vi "integrateCameraEvents.vi"(8 "error in (no error)":errorcluster, 11 "CameraManager in":refnum<class "CameraManager.lvclass">) -> (0 "error out":errorcluster, 3 "CameraManager out":refnum<class "CameraManager.lvclass">)   [LabVIEW 2011, in "iManagement.lvlib" / "CameraManager.lvclass"]
uses:
  CameraManager.lvclass
  CameraManager.lvclass/CameraManager.ctl
  Hal/Channels/Camera/CameraController.lvclass
  Hal/Channels/Camera/CameraEventsManager/CameraEventsManger.lvclass
  Tools/Filing/FileNeologist/FileNeologist.lvclass
  Tools/Filing.lvlib
  Tools/ImageProcessor/BECImageProcessor.lvclass
panel:
  in  "generate error":bool
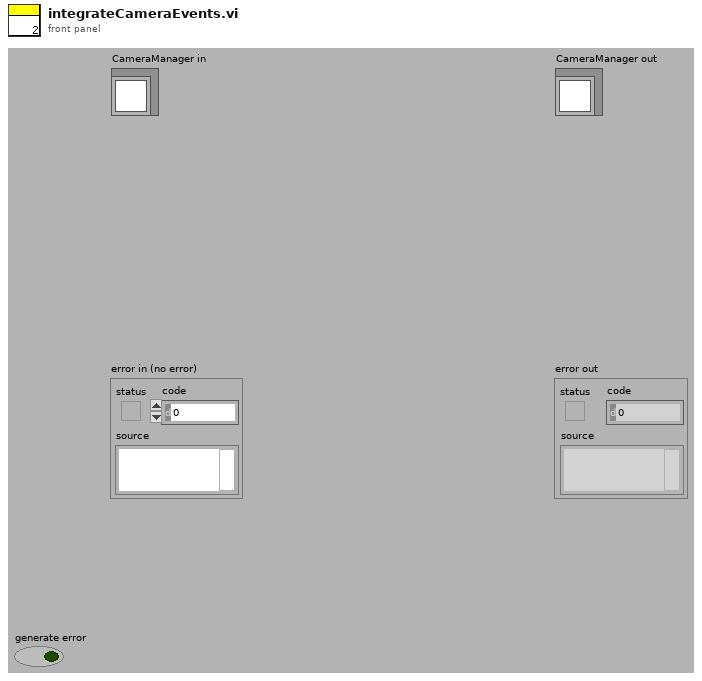
[diagram p1: front panel]
types:
  T1 = cluster{"loadCameraSettingsEvent":refnum<user-event>}
  T2 = cluster{"settingsFrontEndEvents":cluster{"loadSettingsFromPath":refnum<user-event>, "lookUpElementEvent":refnum<user-event>, "saveSettings":refnum<user-event>, "loadSettings":refnum<user-event>, "close":refnum<user-event>, "replaceElement":refnum<user-event>, "findParentNodes":refnum<user-event>, "createNode":refnum<user-event>}, "settingBackEndEvents":cluster{"defaultSettingsPathRequest":refnum<user-event>, "searchResultEvent":refnum<user-event>, "settingsSaved":refnum<user-event>, "settingsLoaded":refnum<user-event>, "foundParentNode":refnum<user-event>}}
  T3 = cluster{"frontEndEvents":cluster{"snapShotEvent":refnum<user-event>, "stopShooting":refnum<user-event>, "userSnapShot":refnum<user-event>}, "backEndEvents":cluster{"picture":refnum<user-event>}}
  T4 = cluster{"snapShotEvent":refnum<user-event>, "stopShooting":refnum<user-event>, "userSnapShot":refnum<user-event>}
  T5 = cluster{"loadSettingsFromPath":refnum<user-event>, "lookUpElementEvent":refnum<user-event>, "saveSettings":refnum<user-event>, "loadSettings":refnum<user-event>, "close":refnum<user-event>, "replaceElement":refnum<user-event>, "findParentNodes":refnum<user-event>, "createNode":refnum<user-event>}
  T6 = cluster{"closeEvent":refnum<user-event>, "temperatureUpdateEvent":refnum<user-event>, "displayErrorEvent":refnum<user-event>, "setPointUpdateEvent":refnum<user-event>}
  T7 = cluster{"Path":path, "atomNumber":dbl, " cloudWidth x":dbl, " cloudWidth z":dbl}
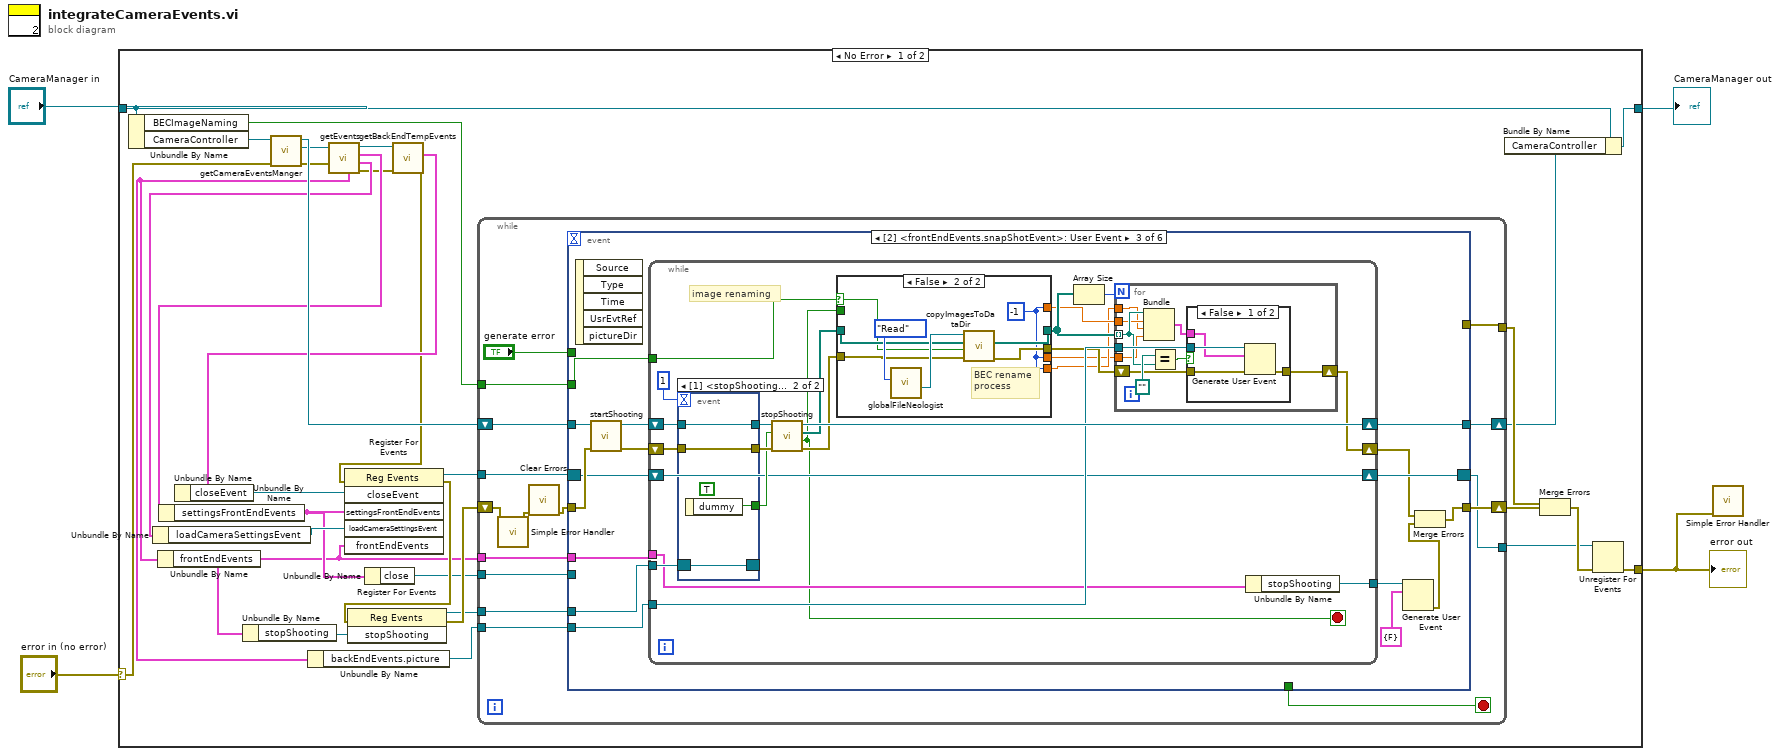
[diagram p0: block diagram]
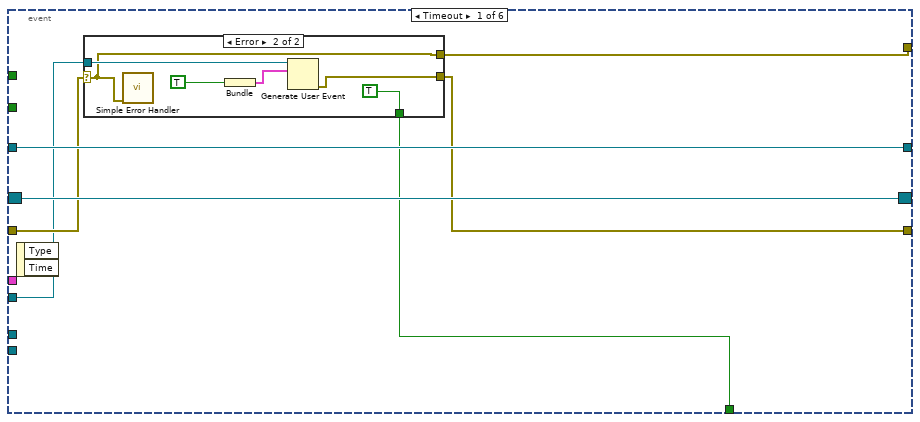
[diagram p2: hidden frame]
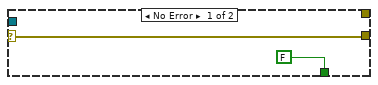
[diagram p3: hidden frame]
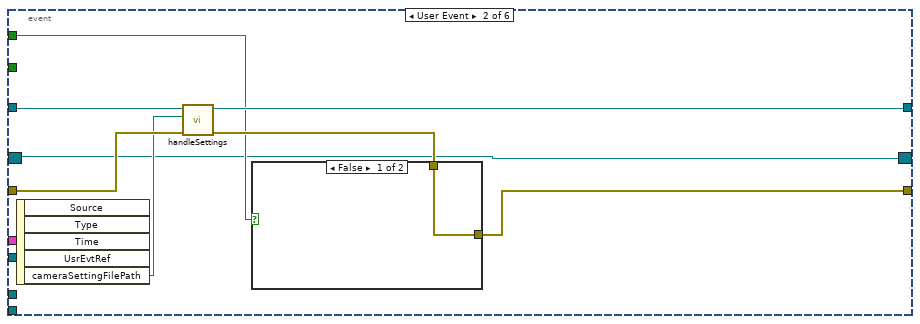
[diagram p4: hidden frame]
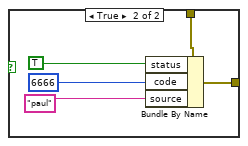
[diagram p5: hidden frame]
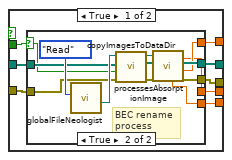
[diagram p6: hidden frame]
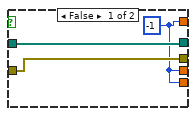
[diagram p7: hidden frame]
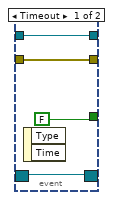
[diagram p9: hidden frame]
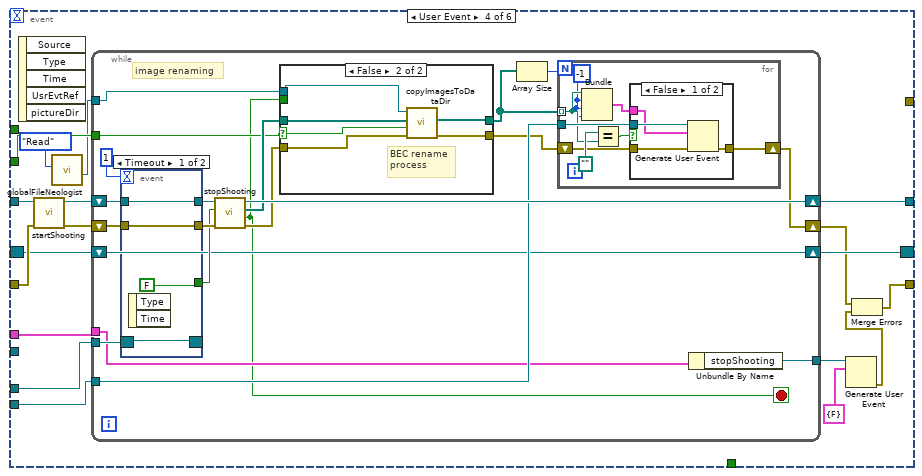
[diagram p10: hidden frame]
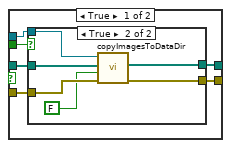
[diagram p11: hidden frame]
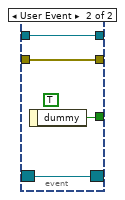
[diagram p14: hidden frame]
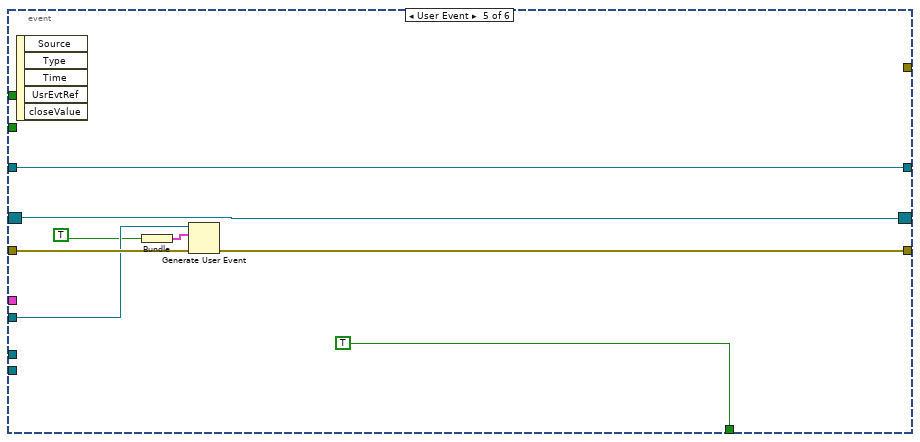
[diagram p15: hidden frame]
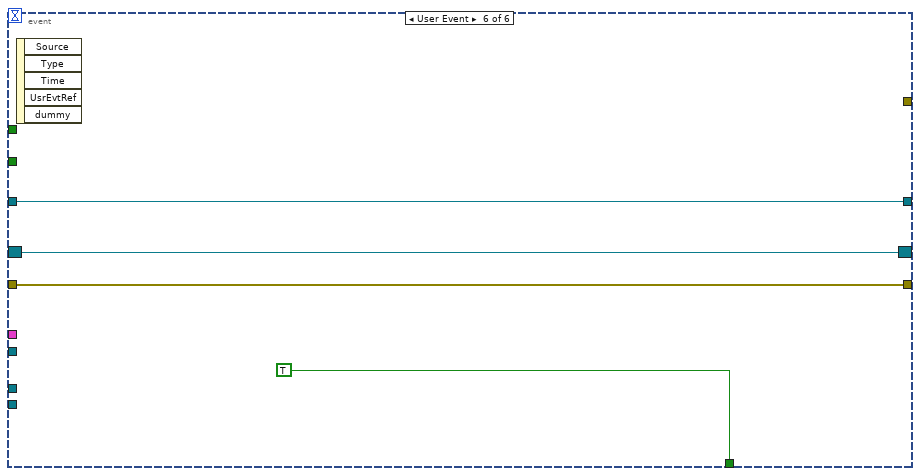
[diagram p16: hidden frame]
diagram:
  n1 = case shown="No Error" "error in (no error)" {
    selector: "error in (no error)" -> [w36 w268]
    tunnel: [w6 w268] -> w1
    tunnel: [w7 w267] -> w2
    tunnel: "CameraManager in" -> [w9 w267]
    frame No Error {
      n2 = Unbundle By Name(w9) -> ("BECImageNaming"=w5:bool, "CameraController"=w35:refnum<class "CameraController.lvclass">)
      n3 = call-dynamic "getCameraEventsManger.vi"("error in (no error)"=w36, "CameraController.lvclass in"=w35) -> ("error out"=w32:errorcluster, "Hardware:Channels.lvlib:CameraEventsManger.lvclass"=w33:refnum<class "CameraEventsManger.lvclass">, "CameraController.lvclass out"=w34:refnum<class "CameraController.lvclass">)  [unwired: 7 in]
      n4 = call-dynamic "getEvents.vi"("error in (no error)"=w32, "CameraEventsManger in"=w33) -> ("error out"=w26:errorcluster, "cameraSettingsEventsRef"=w30:T1, "settingsEvents"=w31:T2, "CameraEventsManger out"=w27:refnum<class "CameraEventsManger.lvclass">, "snapperEvents"=w17:T3)  [unwired: 5 in]
      n5 = Unbundle By Name(w30) -> ("loadCameraSettingsEvent"=w29:refnum<user-event>)
      n6 = Unbundle By Name(w17) -> ("frontEndEvents"=w8:T4)
      n7 = Unbundle By Name(w31) -> ("settingsFrontEndEvents"=w18:T5)
      n8 = Unbundle By Name(w8) -> ("stopShooting"=w28:refnum<user-event>)
      n9 = Unbundle By Name(w17) -> ("backEndEvents.picture"=w16:refnum<user-event>)
      n10 = Unbundle By Name(w18) -> ("close"=w20:refnum<user-event>)
      n11 = call-dynamic "getBackEndTempEvents.vi"("error in (no error)"=w26, "CameraEventsManger.lvclass in"=w27) -> ("error out"=w15:errorcluster, "backEndTempEvents"=w25:T6)  [unwired: 7 in, 1 out]
      n12 = Unbundle By Name(w25) -> ("closeEvent"=w24:refnum<user-event>)
      n13 = register-events(error in=w15, w24, w18, w29, w8) -> (reference out=w23:refnum<event-registration>, error out=w22:errorcluster)  [unwired: 1 in]
      n14 = register-events(error in=w22, w28) -> (reference out=w19:refnum<event-registration>, error out=w21:errorcluster)  [unwired: 1 in]
      n15 = while {
        tunnel: w23 -> [w52]
        shift-right: [w49] -> w10
        shift-left: w34 -> [w50]
        shift-right: [w48] -> w13
        shift-left: w21 -> [w39]
        tunnel: [w47] -> w11
        tunnel: w16 -> [w42]
        tunnel: w19 -> [w46]
        tunnel: w20 -> [w45]
        tunnel: [w44] -> w14
        tunnel: w8 -> [w41]
        tunnel: w5 -> [w40]
        stop <- w51 stop-if-true
        n16 = call <vilib>:"Simple Error Handler.vi"("error in (no error)"=w39) -> ("error out"=w38:errorcluster)  [unwired: 4 in, 4 out]
        n17 = call <vilib>:"Clear Errors.vi"("error in (no error)"=w38) -> ("error out"=w37:errorcluster)  [unwired: 6 in]
        n18 = event shown="[2] <frontEndEvents.snapShotEvent>: User Event" {
          selector: w52 -> [w58 w68 w95 w190 w259 w265]
          dyn-events: [w58 w68 w92 w187 w259 w265] -> w47
          timeout: _ -> [_ _ _ _ _ _]
          tunnel: [w53 _ _ _ TRUE TRUE] -> w51
          tunnel: w50 -> [w59 w75 w97 w192 w262 w264]
          tunnel: [w59 w74 w91 w186 w262 w264] -> w49
          tunnel: w37 -> [w57 w73 w96 w191 w260 w263]
          tunnel: [w56 w70 w84 w175 w261 w263] -> w48
          tunnel: w42 -> [_ _ w90 w185 _ _]
          tunnel: w46 -> [_ _ w89 w184 _ _]
          tunnel: w45 -> [w55 _ _ _ w258 _]
          tunnel: [w54 _ _ _ _ _] -> w44
          tunnel: "generate error" -> [_ w69 _ _ _ _]
          tunnel: w41 -> [_ _ w88 w183 _ _]
          tunnel: w40 -> [_ _ w85 w180 _ _]
          event Timeout {
            n19 = event-data() -> ()  [unwired: 1 in, 2 out]
            n20 = case shown="Error" w57 {
              selector: w57 -> [w61 w62]
              tunnel: [w61 w64] -> w56
              tunnel: w55 -> [_ w65]
              tunnel: [_ w62] -> w54
              tunnel: [FALSE TRUE] -> w53
              frame No Error {
              }
              frame Error {
                n21 = call <vilib>:"Simple Error Handler.vi"("error in (no error)"=w62) -> ()  [unwired: 4 in, 5 out]
                n22 = Bundle(TRUE) -> (w66:cluster{bool})  [unwired: 1 in]
                n23 = Generate User Event(user event=w65, event data cluster=w66) -> (error out=w64:errorcluster)  [unwired: 1 in, 1 out]
              }
            }
          }
          event User Event {
            n24 = event-data() -> ("cameraSettingFilePath"=w72:path)  [unwired: 1 in, 4 out]
            n25 = call-dynamic "handleSettings.vi"("error in (no error)"=w73, "Path"=w72, "CameraController in"=w75) -> ("error out"=w71:errorcluster, "CameraController out"=w74:refnum<class "CameraController.lvclass">)  [unwired: 7 in]
            n26 = case shown="False" w69 {
              tunnel: w71 -> [w76 w81]
              tunnel: [w76 w77] -> w70
              frame False {
              }
              frame True {
                n27 = Bundle By Name(cluster=w81, "status"=TRUE, "code"=6666, "source"="paul") -> (w77:errorcluster)
              }
            }
          }
          event User Event {
            n28 = event-data() -> ()  [unwired: 1 in, 5 out]
            n29 = call-dynamic "startShooting.vi"("error in (no error)"=w96, "CameraController in"=w97) -> ("error out"=w93:errorcluster, "CameraController out"=w94:refnum<class "CameraController.lvclass">)  [unwired: 6 in, 2 out]
            n30 = while {
              shift-right: [w119] -> w91
              shift-left: w94 -> [w120]
              shift-right: [w109] -> w83
              shift-left: w93 -> [w117]
              shift-right: [w111] -> w92
              shift-left: w95 -> [w111]
              tunnel: w90 -> [w113]
              tunnel: w89 -> [w112]
              tunnel: w88 -> [w110]
              tunnel: [w108] -> w87
              tunnel: w85 -> [w102]
              stop <- w101 stop-if-true
              # "image renaming"
              n31 = event shown="[1] <stopShooting>: User Event" {
                selector: w112 -> [w170 w172]
                dyn-events: [w170 w172] -> _
                timeout: 1 -> [_ _]
                tunnel: [w169 w174] -> w118
                tunnel: w120 -> [w169 w174]
                tunnel: w117 -> [w168 w173]
                tunnel: [w168 w173] -> w116
                tunnel: [FALSE w171] -> w114
                event Timeout {
                  n32 = event-data() -> ()  [unwired: 1 in, 2 out]
                }
                event User Event {
                  (unwired) TRUE
                  n33 = event-data() -> ("dummy"=w171:bool)  [unwired: 1 in]
                }
              }
              n34 = call-dynamic "stopShooting.vi"("error in (no error)"=w116, "stop"=w114, "CameraController in"=w118) -> ("error out"=w104:errorcluster, "Stopped"=w101:bool, "Array"=w106:path[], "CameraController out"=w119:refnum<class "CameraController.lvclass">)  [unwired: 5 in]
              n35 = case shown="False" w102 {
                selector: w102 -> [_ w145]
                tunnel: w106 -> [w128 w149]
                tunnel: [w125 w146] -> w105
                tunnel: w104 -> [w127 w148]
                tunnel: [w126 w147] -> w103
                tunnel: w101 -> [w124 _]
                tunnel: [w123 w144] -> w100
                tunnel: [w122 w144] -> w99
                tunnel: [w121 w144] -> w98
                frame True {
                  n36 = case shown="True" w124 {
                    selector: w124 -> [_ w140]
                    tunnel: w128 -> [w131 w141]
                    tunnel: w127 -> [w130 w133]
                    tunnel: [w130 w133] -> w126
                    tunnel: [w131 w137] -> w125
                    tunnel: [w129 w136] -> w123
                    tunnel: [w129 w135] -> w122
                    tunnel: [w129 w134] -> w121
                    frame False {
                      w129 = -1
                    }
                    frame True {
                      # "BEC rename\nprocess"
                      n37 = call "globalFileNeologist.vi"("Action"=enum16{"Write", "Read"}."Read") -> ("FileNeologist out"=w142:refnum<class "FileNeologist.lvclass">)  [unwired: 10 in]
                      n38 = call-dynamic "copyImagesToDataDir.vi"("error in (no error)"=w133, "BECRenaming"=w140, "ImagePaths in"=w141, "FileNeologist in"=w142) -> ("error out"=w139:errorcluster, "ImagePaths out"=w138:path[], "FileNeologist out"=w132:refnum<class "FileNeologist.lvclass">)  [unwired: 5 in]
                      n39 = call "processesAbsorptionImage.vi"("error in (no error)"=w139, "FileNeologist.lvclass out"=w132, "ImagePaths in"=w138) -> ("atomNumber"=w136:dbl, "ImagePaths out"=w137:path[], "cloudWidth x"=w135:dbl, "cloudWidth z"=w134:dbl)  [unwired: 3 in, 2 out]
                    }
                  }
                }
                frame False {
                  w144 = -1
                  # "BEC rename\nprocess"
                  n40 = call "globalFileNeologist.vi"("Action"=enum16{"Write", "Read"}."Read") -> ("FileNeologist out"=w150:refnum<class "FileNeologist.lvclass">)  [unwired: 10 in]
                  n41 = call-dynamic "copyImagesToDataDir.vi"("error in (no error)"=w148, "BECRenaming"=w145, "ImagePaths in"=w149, "FileNeologist in"=w150) -> ("error out"=w147:errorcluster, "ImagePaths out"=w146:path[])  [unwired: 5 in, 1 out]
                }
              }
              n42 = Array Size(array=w105) -> (size(s)=w107:i32)
              n43 = for {
                N: w107 -> [_]
                tunnel: w113 -> [w160]
                shift-right: [w157] -> w109
                shift-left: w103 -> [w158]
                tunnel: w105 -> [w155] mode=indexing
                tunnel: w100 -> [w154]
                tunnel: w99 -> [w153]
                tunnel: w98 -> [w152]
                n44 = Bundle("Path"=w155, "atomNumber"=w154, "cloudWidth x"=w153, "cloudWidth z"=w152) -> (w159:T7)  [unwired: 1 in]
                n45 = Equal?(x=path "", y=w155) -> (x = y?=w156:bool)
                n46 = case shown="False" w156 {
                  tunnel: w160 -> [w165 _]
                  tunnel: w159 -> [w164 _]
                  tunnel: w158 -> [w163 w166]
                  tunnel: [w162 w166] -> w157
                  frame False {
                    n47 = Generate User Event(user event=w165, event data cluster=w164, error in=w163) -> (error out=w162:errorcluster)  [unwired: 1 out]
                  }
                  frame True {
                  }
                }
              }
              n48 = Unbundle By Name(w110) -> ("stopShooting"=w108:refnum<user-event>)
            }
            n49 = Generate User Event(user event=w87, event data cluster=cluster{"dummy":bool} {"dummy"=FALSE} ("event data")) -> (error out=w82:errorcluster)  [unwired: 1 in, 1 out]
            n50 = Merge Errors(w83, w82) -> (w84:errorcluster)
          }
          event User Event {
            n51 = event-data() -> ()  [unwired: 1 in, 5 out]
            n52 = call-dynamic "startShooting.vi"("error in (no error)"=w191, "CameraController in"=w192) -> ("error out"=w188:errorcluster, "CameraController out"=w189:refnum<class "CameraController.lvclass">)  [unwired: 6 in, 2 out]
            n53 = call "globalFileNeologist.vi"("Action"=enum16{"Write", "Read"}."Read") -> ("FileNeologist out"=w178:refnum<class "FileNeologist.lvclass">)  [unwired: 10 in]
            n54 = while {
              shift-right: [w212] -> w186
              shift-left: w189 -> [w213]
              shift-right: [w202] -> w177
              shift-left: w188 -> [w210]
              shift-right: [w204] -> w187
              shift-left: w190 -> [w204]
              tunnel: w185 -> [w206]
              tunnel: w184 -> [w205]
              tunnel: w183 -> [w203]
              tunnel: [w201] -> w182
              tunnel: w180 -> [w195]
              tunnel: w178 -> [w193]
              stop <- w194 stop-if-true
              # "image renaming"
              n55 = event shown="[0] Timeout" {
                selector: w205 -> [w250 w252]
                dyn-events: [w250 w252] -> _
                timeout: 1 -> [_ _]
                tunnel: [w249 w254] -> w211
                tunnel: w213 -> [w249 w254]
                tunnel: w210 -> [w248 w253]
                tunnel: [w248 w253] -> w209
                tunnel: [FALSE w251] -> w207
                event Timeout {
                  n56 = event-data() -> ()  [unwired: 1 in, 2 out]
                }
                event User Event {
                  (unwired) TRUE
                  n57 = event-data() -> ("dummy"=w251:bool)  [unwired: 1 in]
                }
              }
              n58 = call-dynamic "stopShooting.vi"("error in (no error)"=w209, "stop"=w207, "CameraController in"=w211) -> ("error out"=w197:errorcluster, "Stopped"=w194:bool, "Array"=w199:path[], "CameraController out"=w212:refnum<class "CameraController.lvclass">)  [unwired: 5 in]
              n59 = case shown="False" w195 {
                selector: w195 -> [_ w229]
                tunnel: w199 -> [w219 w233]
                tunnel: [w216 w230] -> w198
                tunnel: w197 -> [w218 w232]
                tunnel: [w217 w231] -> w196
                tunnel: w194 -> [w215 _]
                tunnel: w193 -> [w214 w228]
                frame True {
                  n60 = case shown="True" w215 {
                    tunnel: w219 -> [w221 w227]
                    tunnel: w218 -> [w220 w226]
                    tunnel: [w220 w224] -> w217
                    tunnel: [w221 w223] -> w216
                    tunnel: w214 -> [_ w225]
                    frame False {
                    }
                    frame True {
                      n61 = call-dynamic "copyImagesToDataDir.vi"("error in (no error)"=w226, "BECRenaming"=FALSE, "ImagePaths in"=w227, "FileNeologist in"=w225) -> ("error out"=w224:errorcluster, "ImagePaths out"=w223:path[])  [unwired: 5 in, 1 out]
                    }
                  }
                }
                frame False {
                  # "BEC rename\nprocess"
                  n62 = call-dynamic "copyImagesToDataDir.vi"("error in (no error)"=w232, "BECRenaming"=w229, "ImagePaths in"=w233, "FileNeologist in"=w228) -> ("error out"=w231:errorcluster, "ImagePaths out"=w230:path[])  [unwired: 5 in, 1 out]
                }
              }
              n63 = Array Size(array=w198) -> (size(s)=w200:i32)
              n64 = for {
                N: w200 -> [_]
                tunnel: w206 -> [w240]
                shift-right: [w237] -> w202
                shift-left: w196 -> [w238]
                tunnel: w198 -> [w235] mode=indexing
                w234 = -1
                n65 = Bundle("Path"=w235, w234, w234, w234) -> (w239:cluster{"Path":path, i32, i32, i32})  [unwired: 1 in]
                n66 = Equal?(x=path "", y=w235) -> (x = y?=w236:bool)
                n67 = case shown="False" w236 {
                  tunnel: w240 -> [w245 _]
                  tunnel: w239 -> [w242 _]
                  tunnel: w238 -> [w244 w246]
                  tunnel: [w243 w246] -> w237
                  frame False {
                    n68 = Generate User Event(user event=w245, event data cluster=w242, error in=w244) -> (error out=w243:errorcluster)  [unwired: 1 out]
                  }
                  frame True {
                  }
                }
              }
              n69 = Unbundle By Name(w203) -> ("stopShooting"=w201:refnum<user-event>)
            }
            n70 = Generate User Event(user event=w182, event data cluster=cluster{"dummy":bool} {"dummy"=FALSE} ("event data")) -> (error out=w176:errorcluster)  [unwired: 1 in, 1 out]
            n71 = Merge Errors(w177, w176) -> (w175:errorcluster)
          }
          event User Event {
            n72 = event-data() -> ()  [unwired: 1 in, 5 out]
            n73 = Bundle(TRUE) -> (w256:cluster{bool})  [unwired: 1 in]
            n74 = Generate User Event(user event=w258, event data cluster=w256, error in=w260) -> (error out=w261:errorcluster)  [unwired: 1 out]
          }
          event User Event {
            n75 = event-data() -> ()  [unwired: 1 in, 5 out]
          }
        }
      }
      n76 = Bundle By Name(cluster=w9, "CameraController"=w10) -> (w7:refnum<class "CameraManager.lvclass">)
      n77 = Merge Errors(w14, w13) -> (w12:errorcluster)
      n78 = Unregister For Events(event registration refnum=w11, error in=w12) -> (error out=w6:errorcluster)
    }
    frame Error {
    }
  }
  "error out" <- w1
  "CameraManager out" <- w2
  n79 = call <vilib>:"Simple Error Handler.vi"("error in (no error)"=w1) -> ()  [unwired: 4 in, 5 out]
